vi "Send Message.vi"(8 "Error In":errorcluster caption="Fehler (Eingang)", 10 "Nachricht":string, 11 "connection_ID_In":refnum<k5>) -> (0 "Error Out":errorcluster caption="Fehler (Ausgang)", 3 "connection_ID_Out":refnum<k5>)   [LabVIEW 2019, in "Motor Treiber.lvlib"]
uses:
  Motor Treiber.lvlib
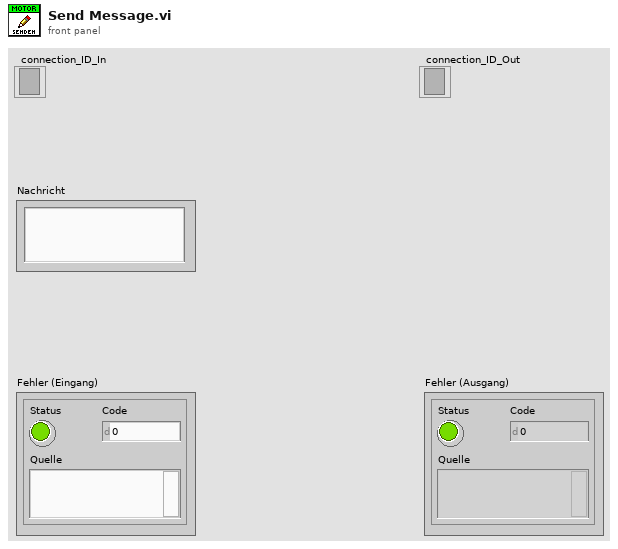
[diagram p1: front panel]
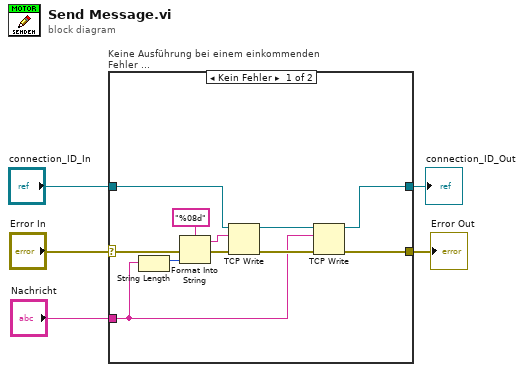
[diagram p0: block diagram]
diagram:
  n1 = case "Keine Ausführung bei einem einkommenden Fehler ..." shown="Kein Fehler" "Error In" {
    selector: "Error In" -> [w16 w18]
    tunnel: [w13 w18] -> w4
    tunnel: "connection_ID_In" -> [w6 w17]
    tunnel: [w14 w17] -> w2
    tunnel: "Nachricht" -> [w8 _]
    frame No Error {
      n2 = String Length(string=w8) -> (length=w11:i32)
      n3 = Format Into String(format string="%08d" ("Format-String"), error in=w16, w11) -> (resulting string=w7:string, error out=w12:errorcluster)  [unwired: 1 in]
      n4 = TCP Write(connection ID=w6, data in=w7, error in (no error)=w12) -> (connection ID out=w9:refnum<k5>, error out=w15:errorcluster)  [unwired: 1 in, 1 out]
      n5 = TCP Write(connection ID=w9, data in=w8, error in (no error)=w15) -> (connection ID out=w14:refnum<k5>, error out=w13:errorcluster)  [unwired: 1 in, 1 out]
    }
    frame Error {
    }
  }
  "Error Out" <- w4
  "connection_ID_Out" <- w2
